vi "Timel series reset globals.vi"(8 "error in (no error)":errorcluster) -> (0 "error out":errorcluster)   [LabVIEW 2020]
uses:
  Global Variables/General Globals.vi
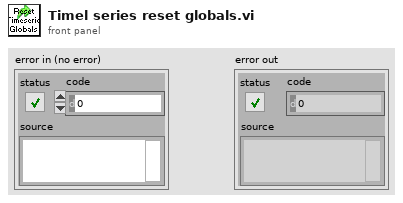
[diagram p1: front panel]
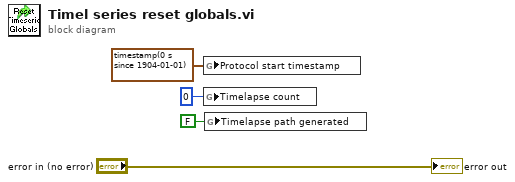
[diagram p0: block diagram]
diagram:
  n1 = global write "General Globals.vi" "Protocol start timestamp"(timestamp(0 s since 1904-01-01) ("Timelapse Start time")) -> ()
  n2 = global write "General Globals.vi" "Timelapse count"(u32 0 ("Timelapse count")) -> ()
  n3 = global write "General Globals.vi" "Timelapse path generated"(FALSE ("Timelapse path generated")) -> ()
  "error out" <- "error in (no error)"
